vi "Translator.Init.vi"(8 "error in":errorcluster, 10 "Language in":string, 11 "Translation folder":path=path "D:/PL_0125_Sapphire_Automation/settings") -> (0 "error out":errorcluster, 2 "Language out":string)   [LabVIEW 2016]
uses:
  Translator.Enums.ctl
  Translator.Message.ctl
  EventLog/EventLog.EventLevelGui.ctl
  Windows/Windows.ExitAction.ctl
  TouchPanel/TouchPanelMonths.ctl
  EventLog/EventLog.EventSource.ctl
  Sequence/Sequence.Step.Status.ctl
  Sequence/Sequence.MainMode.ctl
  Gui/ResultsGui.IncludeOptions.ctl
  Gui/StatisticsGui.TimeSpan.ctl
  Translator.Control.Fglb.Action.vi
  Translator.Global.vi
panel:
  in  "Enums":T1={"Msg"=enum."Quitting", "Level"=enum."ALL", "ExitAction"=enum."Log off from PC", "Month"=enum."January", "Source"=enum."Gui", "TestStatus"=enum."-", "GuiMode"=enum."Process", "ResOptions"=enum."All", "TimeSpan"=enum."All"}
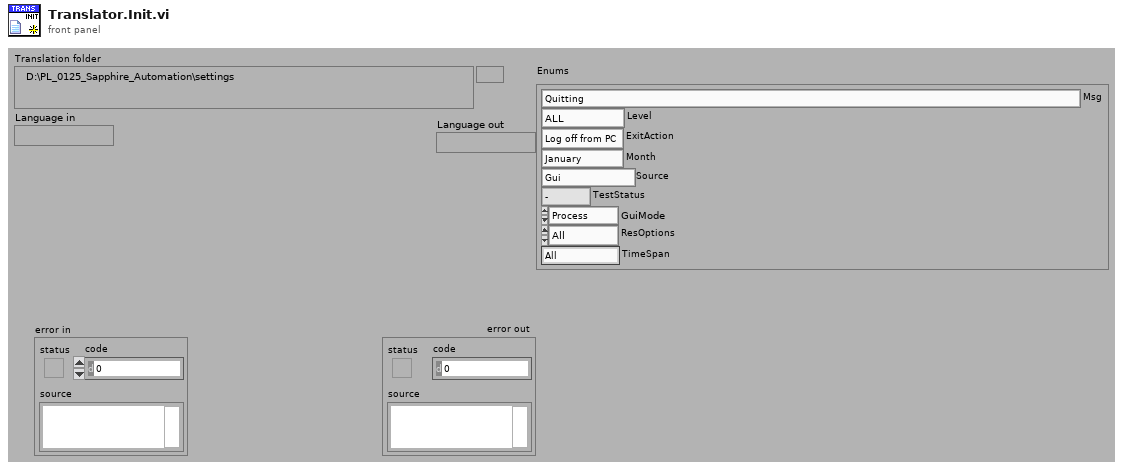
[diagram p1: front panel]
types:
  T1 = typedef "Translator.Enums.ctl" = cluster{"Msg":T2, "Level":T3, "ExitAction":T4, "Month":T5, "Source":T6, "TestStatus":T7, "GuiMode":T8, "ResOptions":T9, "TimeSpan":T10}
  T2 = typedef "Translator.Message.ctl" = enum16{"-", "Event confirmed", "Log out", "Log in", "Shutdown", "Cancel", "Start", "Begin time", "End time", "Duration", "Service Mode", "Ignore Results", "Serial Format", "On", "Off", "OK", "NOK", "NOK %s", "Home", "Work", "Close", "Open", "In progress...", "Missing", "Empty", "Hardware failure", "Initial", "Default", "Total", "Out of range", "Free disk space is below 1GB - contact technician", "Error %d >> %s", "Error %d >> %s >> %s", "Msg %d >> %s", "Laser msg %d %s", "Laser cmd error %s %d", "Laser cmd failed %s", "Laser cmd warning %s", "Laser disconnected", "Laser status %s", "Laser already started", "Laser job unkonwn %s", "Laser job missing %s", "Laser job select failure %s", "Unable to start laser printing (%s)", "Unable to stop laser printing (%s)", "Laser marking aborted", "Laser marking timeout", "Unable to reset Laser Interlock (%s)", "Unable to trigger Laser. Laser not ready (%s)", "Laser job '%s' coordinates not configured", "Starting %s", "Quitting %s", "Configured", "Initializing", "Quitting", "Loading", "Loaded %d results", "Loaded %d events", "Running", "Stopped", "Summary", "Laser", "Do you want to continue?", "Do you want to delete the configuration?", "The configuration is being used by an order. Unable to delete!", "Press confirm button", "Station is not based. Do you want to exit?", "Station requires changeover. Do you want to run the test?", "Test options are not set as default. Do you want to continue?", "Formatting of WabcoNo is disabled. Do you want to continue?", "Product not detected. Do you want to continue?", "Product scan failed. Do you want to continue?", "Calibration", "Log out?", "System", "All", "IDLE", "Translating...%s", "Not found", "Alarm %s", "Run", "Skip", "Abort", "Repeat", "Please wait...", "Database disconnected", "Database disconnected - changeover disabled!", "Login to database successful", "Login to database failed: %d; %s", "Unable to check the product status of reference %d - database disconnected", "Unable to set the product status of reference %d - database disconnected", "Variant file backup %s", "Read variant (%s)", "Result", "Station armed!", "Station requires changeover!", "Select reference number...", "EMERGENCY BUTTON - press Control button", "EMERGENCY DOOR - press Control button", "Resetting Emergency...", "Unable to reset safety circuit - Emergency Button pressed", "Unable to reset safety circuit - Emergency Side Door open", "Station not based", "Station based", "Station not empty", "Station basing...", "No order", "Press Start to begin new order", "Scanning new order", "Order NOK. Correct or scan again", "Order OK. Press Accept", "Order ready", "Revolver incorrect", "Fork incorrect", "Revolver missing", "Revolver empty", "Container missing", "Offline results", "Offline statistics", "Updating statistics %.1f %%", "DMC Configurator", "Door open", "Close the front door", "Press start button", "Done. Open the front door", "Running...", "Running...%.1f %%", "Pause %s", "Pause %s. NOK container missing", "Pause %s. OK container missing", "Pause %s. Revolver empty", "Pause %s. Revolver missing", "Pause %s. Revolver incorrect", "Pause %s. Fork missing", "Pause %s. Fork incorrect", "Pause %s. Too many failures", "Pause %s. Unloading failure", "Pause %s. One slot is not working", "Pause %s. Part order is done. Empty OK container", "Pause %s. Unable to move product to slot", "Pause %s. Unable to move back product pusher", "Pause %s. Unable to lift product", "Pause %s. Unable to move back product lifter", "Pause %s. Unable to move product arm to Work", "Pause %s. Unable to move product arm to NOK", "Pause %s. Unable to move product arm to OK", "Pause %s. Unable to unsuck the NOK product", "Pause %s. Unable to drop the NOK product", "Pause %s. Product OK missing", "Pause %s. Unable to unsuck the OK product", "Pause %s. Unable to drop the OK product", "Stopping...", "File '%s' is missing", "File '%s' is broken", "File '%s' is running", "Log file started (%s)", "Log file ended (%s)", "Log file stopped (%s)", "Log file ignored (%s)", "Log file exported (%s)", "Log file export failed (%s)", "Wrong serial number in log file", "Wrong reference number in log file", "Test steps are missing", "%s = %.3f", "Process param '%s' not found in DB", "Process param '%s' wrong order", "Process param '%s' value %.3f out of limits (%.3f; %.3f)", "Step%d param '%s' not found in DB", "Step%d param '%s' wrong order", "Step%d param '%s' value %.3f out of limits (%.3f; %.3f)", "Step%d EV '%s' not found in DB", "Step%d EV '%s' wrong order", "\"%s\" not found in DB", "\"%s\" wrong order", "\"%s\" value %.3f out of limits (%.3f; %.3f)", "\"%s\" not found in software", "Process init (%s)", "Process started", "Process restarted", "Process run", "Process done", "Process done - remove OK container", "Process aborted", "Process aborted at work", "Process aborted at home", "Process error", "Process error at home", "Process error at work", "Process close", "Process pause", "Process continue", "Process door open", "Process door close", "Process pause at slot %s due to %s", "Select plate from the order to process", "Do you want to start the process?", "Do you want to continue the process?", "There is unfinished order. Do you want to put the new order?", "Product %s %d OK", "Product %s %d NOK", "Unable to unload the slot %s. Product missing in the slot", "Unable to unload the slot %s. Product already in the arm", "Unable to accept the product as OK. Product missing in slot %s", "Unable to accept the product as OK. Product could not drop into the container at slot %s", "Unable to accept the product as NOK. Product could not drop into the container at slot %s", "Scan failed. Error %s", "Scan failed. Scanner disconnected", "Scan failed. Wrong Wabco number %d, limit (%d,%d)", "Scan failed. Wrong serial number %d, limit (%d,%d)", "Scan failed. Wrong date %d, limit (%d,%d)", "Scan failed. Wrong product wabco number %d (expected %d)", "Scan failed. Wrong product serial number %d (expected > 0)", "Scan OK %s", "Scan failed. Unable to determine table position (%s)", "Scan failed. Timeout", "Tune failed. Scanner disconnected", "Tune failed. Timeout", "%s = %d", "%s = %d->%d", "Unable to set %s = %.2f - Air Pressure Inside off", "Unable to set digital output '%s' = %d", "Unable to activate air pressure inside - timeout", "Unable to activate air pressure inside - aborted", "Unable to switch on Air Main Valve - Air Pressure Inlet off", "Unable to switch on Air Main Valve - Door open", "Unable to switch off Air Main Valve - timeout", "Unable to switch off Air Main Valve - aborted", "Unable to rotate Table - timeout", "Unable to rotate Table - aborted", "Unable to rotate Table - Product Move not in Home position", "Unable to rotate Table - Air Pressure Inside off", "Unable to rotate Table - Product Lift A not in Home position", "Unable to rotate Table - Product Lift B not in Home position", "Unable to rotate Table - unlock before movement timeout", "Unable to rotate Table - lock after movement timeout", "Unable to move Table Lock to %s position - timeout", "Unable to move Table Lock to %s position - aborted", "Unable to move Table Lock to %s position - Air Pressure Inside off", "Unable to move Table Lock to %s position - Table not in position", "Unable to move Product Lift A to %s position - timeout", "Unable to move Product Lift B to %s position - timeout", "Unable to move Product Lift A to %s position - aborted", "Unable to move Product Lift B to %s position - aborted", "Unable to move Product Lift A to %s position - Air Pressure Inside off", "Unable to move Product Lift B to %s position - Air Pressure Inside off", "Unable to move Product Lift A to %s position - Table not locked", "Unable to move Product Lift B to %s position - Table not locked", "Unable to move Product Lift A to %s position - Product Arm not in Work position", "Unable to move Product Lift B to %s position - Product Arm not in Work position", "Unable to set Product Suction Gripper %s to %s - timeout", "Unable to set Product Suction Gripper %s to %s - aborted", "Unable to set Product Suction Gripper %s to %s - Air Pressure Inside off", "Unable to set Product Suction Gripper %s to %s - Table slot unkown", "Unable to move Product Arm to %s position - timeout", "Unable to move Product Arm to %s position - aborted", "Unable to move Product Arm to %s position - Air Pressure Inside off", "Unable to move Product Arm to %s position - Product Lift A not in Home position", "Unable to move Product Arm to %s position - Product Lift B not in Home position", "Unable to move Product to %s position - timeout", "Unable to move Product to %s position - aborted", "Unable to move Product to %s position - Air Pressure Inside off", "Unable to move Product to %s position - Table not in position"}
  T3 = typedef "EventLog.EventLevelGui.ctl" = enum16{"ALL", "Debug", "Info", "Warning", "Error"}
  T4 = typedef "Windows.ExitAction.ctl" = enum16{"Log off from PC", "Shut Down PC", "Reboot PC", "Close Program"}
  T5 = typedef "TouchPanelMonths.ctl" = enum16{"January", "February", "March", "April", "May", "June", "July", "August", "September", "October", "November", "December"}
  T6 = typedef "EventLog.EventSource.ctl" = enum16{"All", "Gui", "Ref", "File", "Arch", "Seq", "CPX", "DB", "Laser", "Scan.P", "Scan.O"}
  T7 = typedef "Sequence.Step.Status.ctl" = enum16{"-", "Pending", "Running", "Skipped", "Passed", "Failed", "Done", "Error", "Aborted", "Stopped"}
  T8 = typedef "Sequence.MainMode.ctl" = enum16{"Process", "Base", "Order", "Manual", "Logs", "Results", "Stats", "DMC Config"}
  T9 = typedef "ResultsGui.IncludeOptions.ctl" = enum16{"All", "Temporary", "Exported", "Error"}
  T10 = typedef "StatisticsGui.TimeSpan.ctl" = enum16{"All", "Shift(s)", "Hour(s)", "Day(s)", "Week(s)", "Month(s)", "Custom"}
  T11 = typedef "Translator.Control.Fglb.Action.vi" = enum16{"init", "set", "get", "clear"}
  T12 = enum32{"invalid app kind", "Development System", "Run Time System", "Student Edition", "Embedded LabVIEW", "Evaluation", "Custom"}
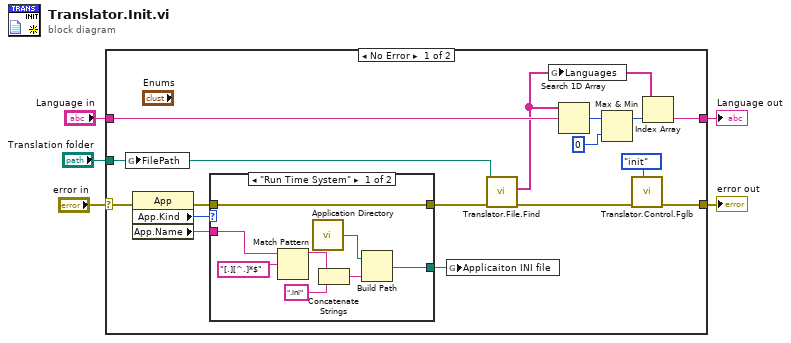
[diagram p0: block diagram]
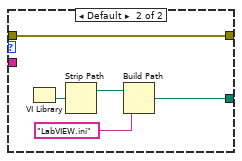
[diagram p2: hidden frame]
diagram:
  n1 = case shown="No Error" "error in" {
    selector: "error in" -> [w19 w36]
    tunnel: [w8 w36] -> w5
    tunnel: "Translation folder" -> [w6 _]
    tunnel: "Language in" -> [w13 w35]
    tunnel: [w11 w35] -> w1
    frame No Error {
      n2 = global write "Translator.Global.vi" "FilePath"(w6) -> ()
      n3 = property class="App"(error in=w19) -> (error out=w21:errorcluster, "App.Kind"=w20:T12, "App.Name"=w10:string)  [unwired: 1 in, 1 out]
      n4 = case shown="\"Run Time System\"" w20 {
        tunnel: [w29 w34] -> w18
        tunnel: w21 -> [w29 w34]
        tunnel: [w27 w30] -> w14
        tunnel: w10 -> [w25 _]
        frame "Run Time System" {
          n5 = Match Pattern(string=w25, regular expression="[.][^.]*$") -> (before substring=w24:string)  [unwired: 4 out]
          n6 = call <vilib>:"Application Directory.vi"() -> ("Application Directory"=w28:path)
          n7 = Concatenate Strings(w24, ".ini" ("string")) -> (w22:string)
          n8 = Build Path(base path=w28, name or relative path=w22) -> (appended path=w27:path)
        }
        frame Default {
          n9 = VI Library() -> (path=w33:path)
          n10 = Strip Path(path=w33) -> (stripped path=w32:path)  [unwired: 1 out]
          n11 = Build Path(base path=w32, name or relative path="LabVIEW.ini") -> (appended path=w30:path)
        }
      }
      n12 = global write "Translator.Global.vi" "Applicaiton INI file"(w14) -> ()
      n13 = call "Translator.File.Find.vi"("error in"=w18, "Translation folder"=w6) -> ("error out"=w9:errorcluster, "Languages"=w12:string[])  [unwired: 8 in]
      n14 = global write "Translator.Global.vi" "Languages"(w12) -> ()
      n15 = Search 1D Array(1D array=w12, element=w13) -> (index of element=w15:i32)  [unwired: 1 in]
      n16 = Max & Min(x=w15, y=0) -> (max(x,y)=w16:i32)  [unwired: 1 out]
      n17 = call "Translator.Control.Fglb.vi"("Action"=Translator.Control.Fglb.Action.vi."init", "error in (no error)"=w9) -> ("error out"=w8:errorcluster)  [unwired: 8 in, 1 out]
      n18 = Index Array(array=w12, index=w16) -> (element=w11:string)
    }
    frame Error {
    }
  }
  "error out" <- w5
  "Language out" <- w1
